vi "ObtainEvents.vi"(7 "Set? (f)":bool, 8 "error in (no error)":errorcluster) -> (0 "error out":errorcluster, 3 "clEvent":T1)   [LabVIEW 2014, in "FgenPlugins.lvlib" / "DaqMx_Single.lvclass"]
uses:
  DaqMx_Single.lvclass
  clEvents.ctl
  EventType.ctl
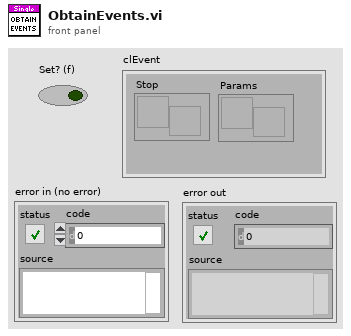
[diagram p1: front panel]
types:
  T1 = typedef "FgenPlugins.lvlib/DaqMx_Single.lvclass/clEvents.ctl" = cluster{"Stop":refnum<user-event>, "Params":refnum<user-event>}
  T2 = typedef "clEvents.ctl" = cluster{"Stop":refnum<user-event>, "Params":refnum<user-event>}
  T3 = typedef "FgenPlugins.lvlib/DaqMx_Single.lvclass/EventType.ctl" = cluster{"Data":variant}
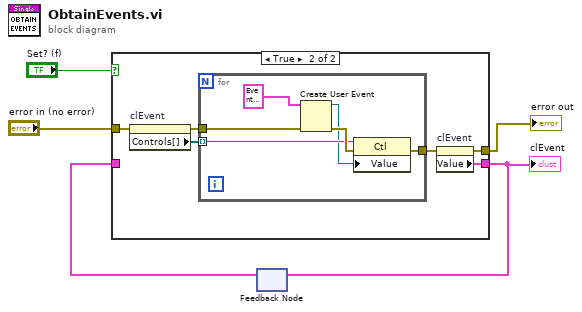
[diagram p0: block diagram]
diagram:
  n1 = feedback #1() -> (w4:T2)  [unwired: 1 in]
  n2 = case shown="True" "Set? (f)" {
    tunnel: [w7 w10] -> w3
    tunnel: w4 -> [w7 _]
    tunnel: "error in (no error)" -> [w6 w9]
    tunnel: [w6 w8] -> w1
    frame False {
    }
    frame True {
      n3 = property on="clEvent" class="Clust (strict)"(error in=w9) -> (error out=w12:errorcluster, "Controls[]"=w13:refnum<vi>[])  [unwired: 1 in, 1 out]
      n4 = for {
        tunnel: [w18] -> w11
        tunnel: w13 -> [w17] mode=indexing
        tunnel: w12 -> [w16]
        n5 = Create User Event(user event datatype=T3 {"Data"=variant} ("EventType"), error in=w16) -> (user event=w15:refnum<user-event>, error out=w19:errorcluster)
        n6 = property class="Ctl"(reference=w17, error in=w19, "Value"=w15) -> (error out=w18:errorcluster)  [unwired: 1 out]
      }
      n7 = property on="clEvent" class="Clust (strict)"(error in=w11) -> (error out=w8:errorcluster, "Value"=w10:T2)  [unwired: 1 in, 1 out]
    }
  }
  "clEvent" <- w3
  "error out" <- w1
  n8 = feedback-in #1(w3) -> ()
